vi "WB_import_convert255_separate_sub_양수.vi"(0 "weights&Biases_cvs_file path":path=path "C:/Users/박원일/NEPL Dropbox/연구실 공용/뉴로모픽 과제/weights/weights_f_93.csv", 2 "format (%.3f)":string="%.3f") -> (3 "max value":dbl, 4 "min value":dbl, 5 "Weights & Biases":dbl[][](array[numeric]), 6 "Weights":i64[][](array[numeric]), 7 "Biases":i64[](array[numeric]), 8 "No.Input":i32, 9 "No.Output":i32)   [LabVIEW 2021]
uses:
  <vilib>/Utility/file.llb/Read Delimited Spreadsheet (DBL).vi
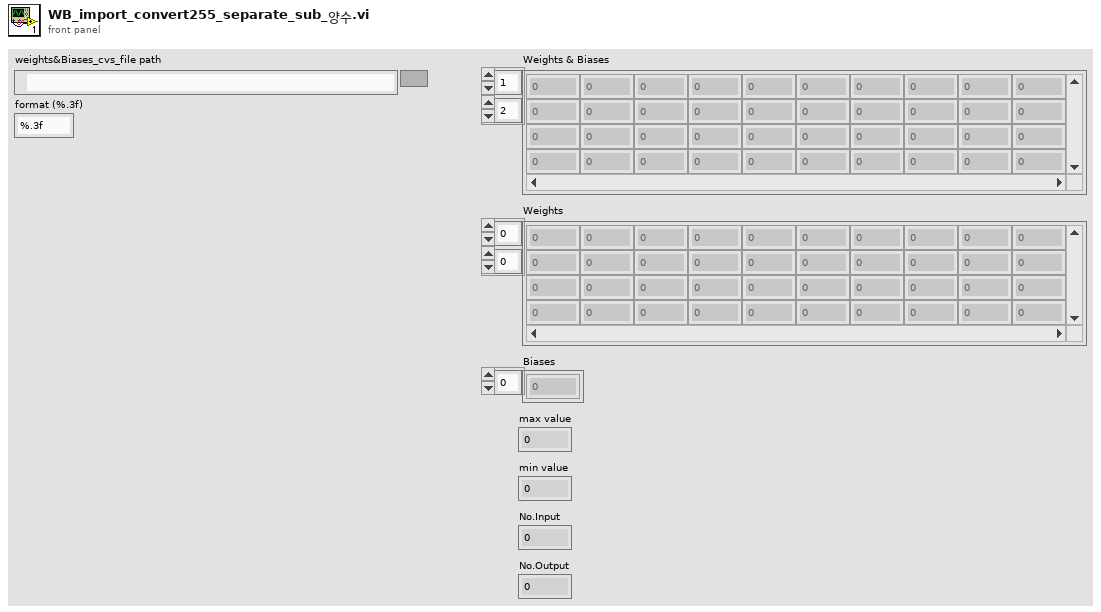
[diagram p1: front panel]
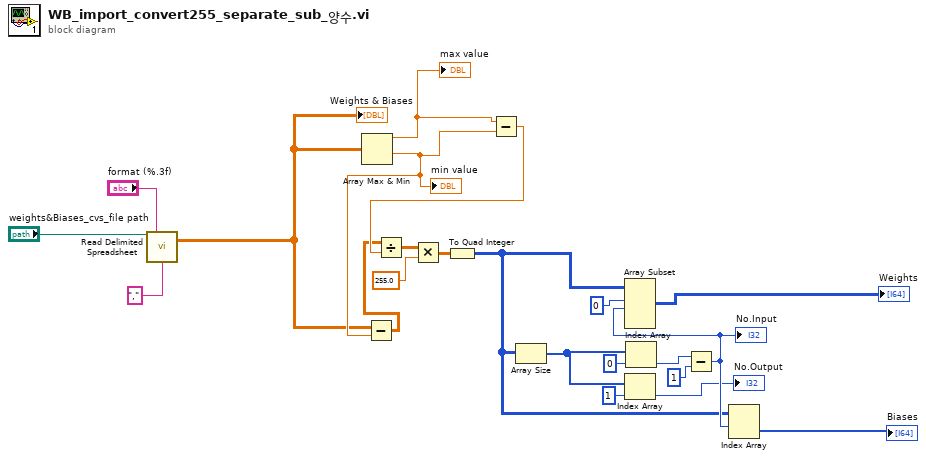
[diagram p0: block diagram]
diagram:
  n1 = call-poly <vilib>:"Read Delimited Spreadsheet.vi"("file path (dialog if empty)"="weights&Biases_cvs_file path", "format (%.3f)"="format (%.3f)", "delimiter (\\t)"="," ("delimiter (\\t)")) -> ("all rows"=w2:dbl[][])  [unwired: 7 in, 5 out]
  "Weights & Biases" <- w2
  n2 = Array Max & Min(array=w2) -> (max value=w5:dbl, min value=w3:dbl)  [unwired: 2 out]
  "max value" <- w5
  "min value" <- w3
  n3 = Subtract(x=w2, y=w3) -> (x-y=w1:dbl[][])
  n4 = Subtract(x=w5, y=w3) -> (x-y=w4:dbl)
  n5 = Divide(x=w1, y=w4) -> (x/y=w8:dbl[][])
  n6 = Multiply(x=w8, y=255.0) -> (x*y=w7:dbl[][])
  n7 = To Quad Integer(1:w7) -> (0:w6:i64[][])
  n8 = Array Size(array=w6) -> (size(s)=w17:i32[])
  n9 = Index Array(array=w17, index=1 ("인덱스")) -> (element=→"No.Output":i32)
  n10 = Index Array(array=w17, index=0 ("인덱스")) -> (element=w15:i32)
  n11 = Subtract(x=w15, y=1) -> (x-y=w13:i32)
  "No.Input" <- w13
  n12 = Array Subset(array=w6, index (row)=0 ("인덱스"), length (row)=w13) -> (→"Weights":i64[][])  [unwired: 2 in]
  n13 = Index Array(array=w6, index (row)=w13) -> (element=→"Biases":i64[])  [unwired: 1 in]
